vi "Calculate Possible Combinations.vi"(10 "Reasonable Search Amount":i32=1000, 11 "Character Position Possible Letters":T1) -> (2 "Reasonable Search Amount?":bool, 3 "Possible Combinations":i32)   [LabVIEW 2025, in "WordleSolver.lvlib"]
uses:
  WordleSolver.lvlib
  Controls/Character Position Possible Letters.ctl
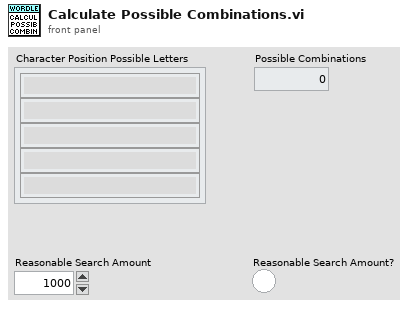
[diagram p1: front panel]
types:
  T1 = typedef "Character Position Possible Letters.ctl" = string[]
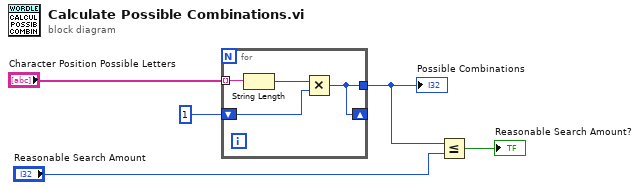
[diagram p0: block diagram]
diagram:
  n1 = for {
    tunnel: "Character Position Possible Letters" -> [w9] mode=indexing
    tunnel: [w6] -> w4
    shift-right: [w6] -> _
    shift-left: 1 -> [w7]
    n2 = String Length(string=w9) -> (length=w8:i32)
    n3 = Multiply(x=w8, y=w7) -> (x*y=w6:i32)
  }
  "Possible Combinations" <- w4
  n4 = Less Or Equal?(x=w4, y="Reasonable Search Amount") -> (x <= y?=→"Reasonable Search Amount?":bool)
